vi "FindGObj.vi"(1 "Name":string, 2 "VI":refnum<vi>) -> (0 "GObj":refnum<vi>)   [LabVIEW 2014]
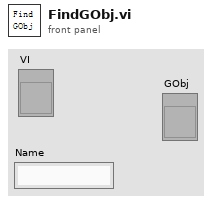
[diagram p1: front panel]
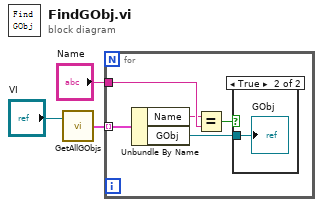
[diagram p0: block diagram]
diagram:
  n1 = call "GetAllGObjs.vi"("VI"="VI") -> ("GObjs"=w2:cluster{"Name":string, "GObj":refnum<vi>}[])  [unwired: 1 in]
  n2 = for {
    tunnel: w2 -> [w6] mode=indexing
    tunnel: "Name" -> [w8]
    n3 = Unbundle By Name(w6) -> ("Name"=w5:string, "GObj"=w4:refnum<vi>)
    n4 = Equal?(x=w5, y=w8) -> (x = y?=w7:bool)
    n5 = case shown="True" w7 {
      tunnel: w4 -> [_ w9]
      frame False {
      }
      frame True {
        "GObj" <- w9
      }
    }
  }
